vi "Write timeout ms (wait forever_ -1).vi"(8 "error in (no error)":errorcluster, 10 "timeout ms (wait forever: -1)":i32=-1, 11 "WebSocket Listener Actor in":refnum<class "WebSocket Service.lvclass">) -> (0 "error out":errorcluster, 3 "WebSocket Listener Actor out":refnum<class "WebSocket Service.lvclass">)   [LabVIEW 2016, in "WebSocket Actors.lvlib" / "WebSocket Service.lvclass"]
uses:
  WebSocket Service.lvclass
  WebSocket Service.lvclass/WebSocket Service.ctl
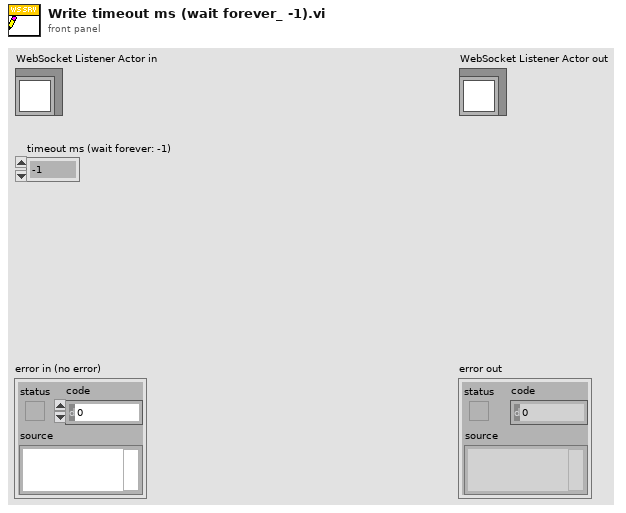
[diagram p1: front panel]
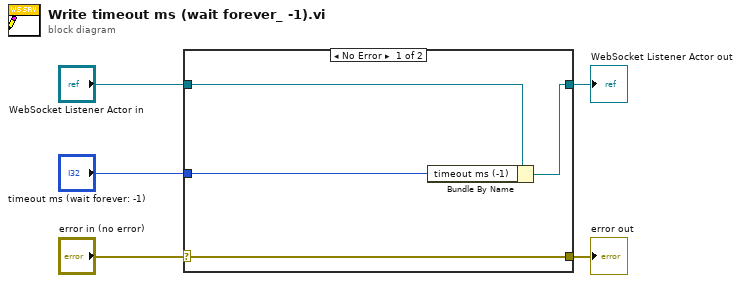
[diagram p0: block diagram]
diagram:
  n1 = case shown="No Error" "error in (no error)" {
    selector: "error in (no error)" -> [w9 w10]
    tunnel: [w9 w10] -> w4
    tunnel: [w7 w11] -> w2
    tunnel: "WebSocket Listener Actor in" -> [w8 w11]
    tunnel: "timeout ms (wait forever: -1)" -> [w6 _]
    frame No Error {
      n2 = Bundle By Name(cluster=w8, "timeout ms (-1)"=w6) -> (w7:refnum<class "WebSocket Service.lvclass">)
    }
    frame Error {
    }
  }
  "error out" <- w4
  "WebSocket Listener Actor out" <- w2
